vi "Node v1.vi"() -> ()   [LabVIEW 2016]
uses:
  PXImc Router/Controls/Node Data.ctl
  <vilib>/NI Veristand/VeriStand Data/Byte Buffer/Byte Buffer.lvclass
  PXImc Router/Controls/Node/Node - PXImc Parameters.ctl
  PXImc Router/Controls/Node/Node - Writer Data.ctl
  PXImc Router/Controls/Node/Node Ch Properties.ctl
  PXImc Router/Controls/Data Type.ctl
  PXImc Router/Controls/Node/Node - Readers Data.ctl
  PXImc Router/Controls/Node/Node - Reader Data.ctl
  <vilib>/Utility/error.llb/DialogType.ctl
  PXImc Router/VIs/Node/Node - Globals.vi
  PXImc Router/PXImc Router.lvlib
panel:
  in  "Node 2 Data In":T1
  out "Reader Node 2":T8(graph)
  out "Node 2 - Reader Ch":dbl[](array[numeric])
  in  "index 2":i32
  in  "length 2":i32
  out "Writer Node 2":T8(graph)={"[0]"=1.0, "[1]"=2.0, "[2]"=3.0, "[3]"=4.0, "[4]"=5.0, "[5]"=0.0, "[6]"=0.0, "[7]"=0.0, "[8]"=0.0}
  in  "Node 2 - Writer Ch":dbl[](array[numeric])
  in  "length":i32
  in  "index":i32
  out "Node 1 - Reader Ch":dbl[](array[numeric])
  in  "Node 1 Data In":T1
  in  "Node 1 - Writer Ch":dbl[](array[numeric])
  in  "stop":bool
  out "Writer Node 1":T8(graph)={"[0]"=1.0, "[1]"=2.0, "[2]"=3.0, "[3]"=4.0, "[4]"=5.0, "[5]"=0.0, "[6]"=0.0, "[7]"=0.0, "[8]"=0.0}
  out "Reader Node 1":T8(graph)
  # "Node 1"
  # "Node 2"
  # "Node 2 => Node 1"
  # "Node 1 => Node 2"
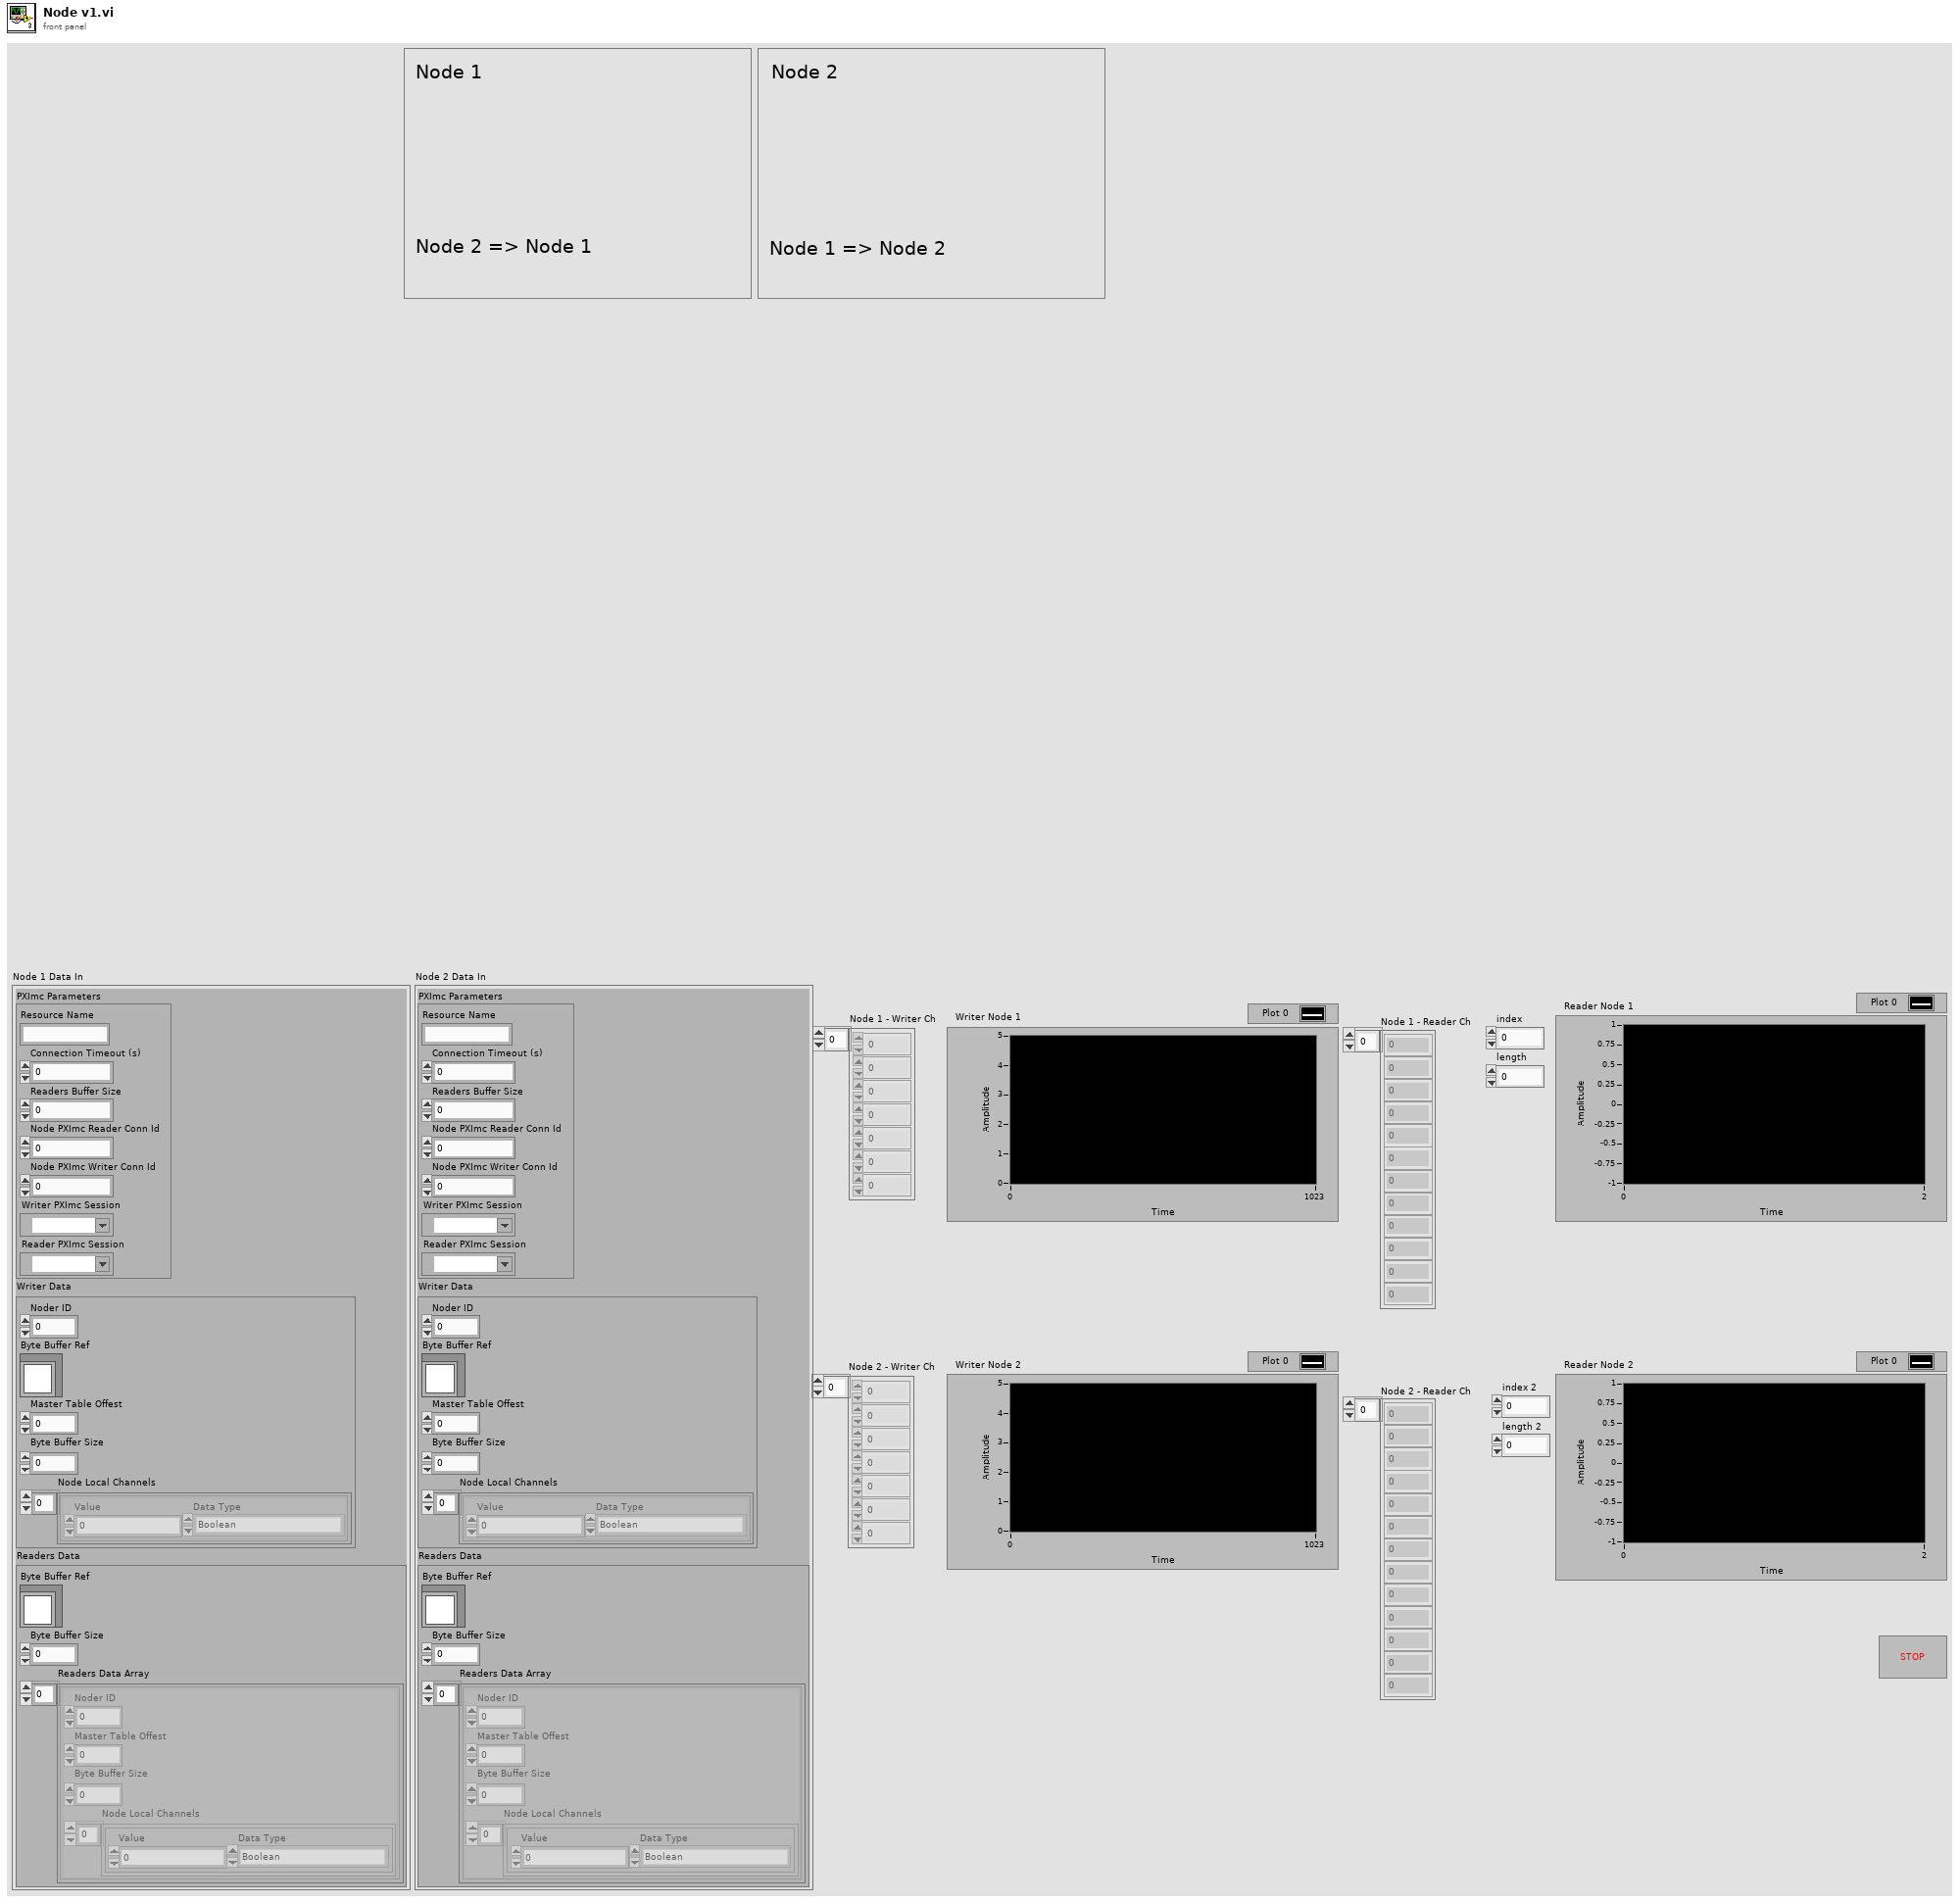
[diagram p1: front panel]
types:
  T1 = typedef "PXImc Router.lvlib/Node Data.ctl" = cluster{"PXImc Parameters":T2, "Writer Data":T3, "Readers Data":T6}
  T2 = typedef "PXImc Router.lvlib/Node - PXImc Parameters.ctl" = cluster{"Resource Name":string, "Connection Timeout (s)":dbl, "Readers Buffer Size":u64, "Node PXImc Reader Conn Id":u16, "Node PXImc Writer Conn Id":u16, "Writer PXImc Session":refnum<k21>, "Reader PXImc Session":refnum<k21>}
  T3 = typedef "PXImc Router.lvlib/Node - Writer Data.ctl" = cluster{"Noder ID":u32, "Byte Buffer Ref":refnum<class "Byte Buffer.lvclass">, "Master Table Offest":u32, "Byte Buffer Size":u32, "Node Local Channels":T4[]}
  T4 = typedef "PXImc Router.lvlib/Node Ch Properties.ctl" = cluster{"Value":dbl, "Data Type":T5}
  T5 = typedef "PXImc Router.lvlib/Data Type.ctl" = enum16{"Boolean", "SGL", "DBL", "I8", "I16", "I32", "I64", "U8", "U16", "U32", "U64"}
  T6 = typedef "PXImc Router.lvlib/Node - Readers Data.ctl" = cluster{"Byte Buffer Ref":refnum<class "Byte Buffer.lvclass">, "Byte Buffer Size":u64, "Readers Data Array":T7[]}
  T7 = typedef "PXImc Router.lvlib/Node - Reader Data.ctl" = cluster{"Noder ID":u32, "Master Table Offest":u32, "Byte Buffer Size":u64, "Node Local Channels":T4[]}
  T8 = cluster{"[0]":dbl, "[1]":dbl, "[2]":dbl, "[3]":dbl, "[4]":dbl, "[5]":dbl, "[6]":dbl, "[7]":dbl, "[8]":dbl}
  T9 = typedef "DialogType.ctl" = u16
  T10 = cluster{"Node 1 - Writer Ch[0]":dbl, "Node 1 - Writer Ch[1]":dbl, "Node 1 - Writer Ch[2]":dbl, "Node 1 - Writer Ch[3]":dbl, "Node 1 - Writer Ch[4]":dbl, "Node 1 - Writer Ch[5]":dbl, "Node 1 - Writer Ch[6]":dbl, "Node 1 - Writer Ch[7]":dbl, "Node 1 - Writer Ch[8]":dbl}
  T11 = cluster{"Node 2 - Writer Ch[0]":dbl, "Node 2 - Writer Ch[1]":dbl, "Node 2 - Writer Ch[2]":dbl, "Node 2 - Writer Ch[3]":dbl, "Node 2 - Writer Ch[4]":dbl, "Node 2 - Writer Ch[5]":dbl, "Node 2 - Writer Ch[6]":dbl, "Node 2 - Writer Ch[7]":dbl, "Node 2 - Writer Ch[8]":dbl}
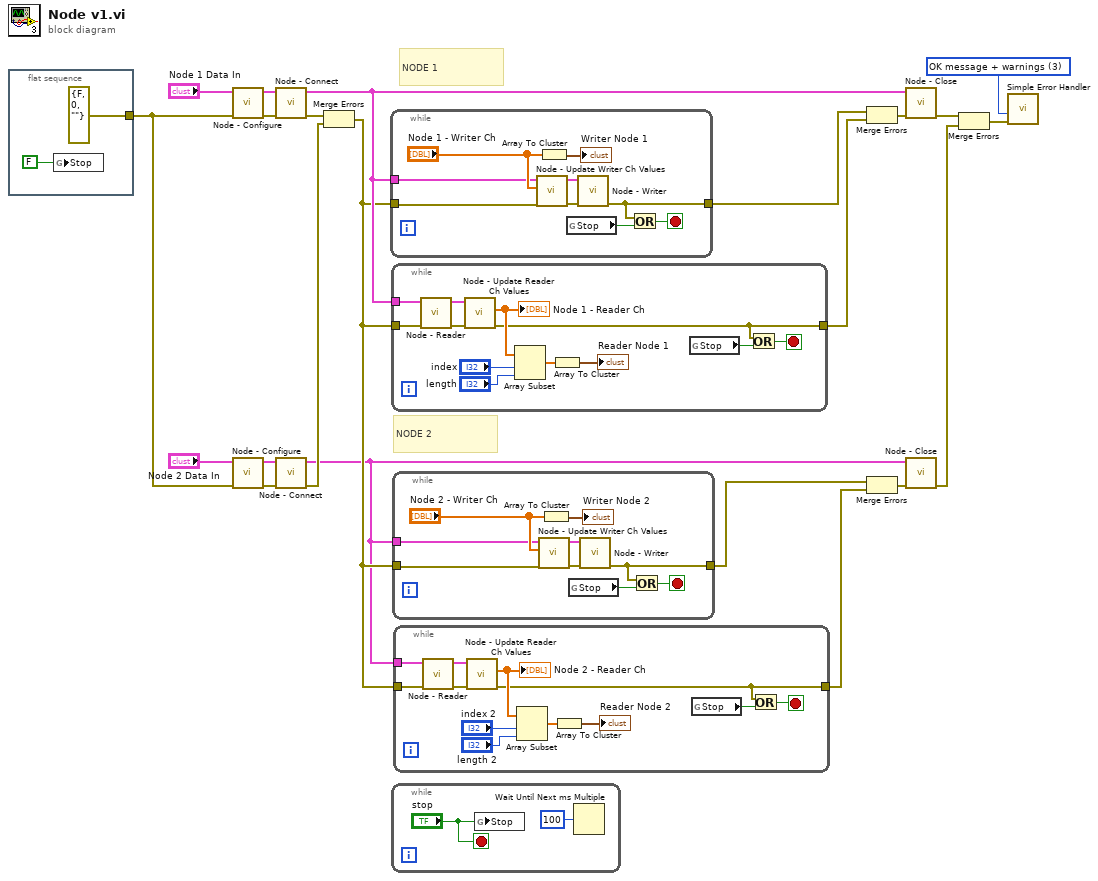
[diagram p0: block diagram]
diagram:
  w22 = T9 3 items=["no dialog", "OK message", "continue or stop message", "OK message + warnings", "continue/stop + warnings"] ("type of dialog (OK msg:1)")
  # "NODE 2"
  # "NODE 1"
  n1 = flat-sequence {
    tunnel: [errorcluster {"status"=FALSE, "code"=0, "source"=""} ("error constant")] -> w6
    frame #0 {
      n2 = global write "Node - Globals.vi" "Stop"(FALSE ("Stopped")) -> ()
    }
  }
  n3 = call "Node - Configure.vi"("error in (no error)"=w6, "Node Data In"="Node 1 Data In") -> ("error out"=w18:errorcluster, "Node Data Out"=w19:T1)  [unwired: 8 in]
  n4 = call "Node - Configure.vi"("error in (no error)"=w6, "Node Data In"="Node 2 Data In") -> ("error out"=w10:errorcluster, "Node Data Out"=w9:T1)  [unwired: 8 in]
  n5 = call "Node - Connect.vi"("error in (no error)"=w18, "Node Data In"=w19) -> ("error out"=w17:errorcluster, "Node Data Out"=w14:T1)  [unwired: 8 in]
  n6 = call "Node - Connect.vi"("error in (no error)"=w10, "Node Data In"=w9) -> ("error out"=w7:errorcluster, "Node Data Out"=w4:T1)  [unwired: 8 in]
  n7 = Merge Errors(w17, w7) -> (w8:errorcluster)
  n8 = while {
    tunnel: w14 -> [w28]
    tunnel: w8 -> [w27]
    tunnel: [w31] -> w21
    stop <- w32 stop-if-true
    n9 = call "Node - Update Writer Ch Values.vi"("error in (no error)"=w27, "Writer Channels In"="Node 1 - Writer Ch", "Node Data In"=w28) -> ("error out"=w25:errorcluster, "Node Data Out"=w26:T1)  [unwired: 7 in]
    n10 = Array To Cluster(array="Node 1 - Writer Ch") -> (cluster=→"Writer Node 1":T10)
    n11 = global read "Node - Globals.vi" "Stop"() -> (w33:bool)
    n12 = call "Node - Writer.vi"("error in (no error)"=w25, "Node Data In"=w26) -> ("error out"=w31:errorcluster)  [unwired: 8 in, 1 out]
    n13 = Or(x=w31, y=w33) -> (x .or. y?=w32:bool)
  }
  n14 = while {
    tunnel: w14 -> [w41]
    tunnel: w8 -> [w45]
    tunnel: [w34] -> w20
    stop <- w43 stop-if-true
    n15 = call "Node - Reader.vi"("error in (no error)"=w45, "Node Data In"=w41) -> ("error out"=w39:errorcluster, "Node Data Out"=w40:T1)  [unwired: 8 in]
    n16 = call "Node - Update Reader Ch Values.vi"("error in (no error)"=w39, "Node Data In"=w40) -> ("error out"=w34:errorcluster, "Reader Ch Out"=w37:dbl[])  [unwired: 7 in, 1 out]
    "Node 1 - Reader Ch" <- w37
    n17 = Array Subset(array=w37, index="index", length="length") -> (w38:dbl[])
    n18 = Array To Cluster(array=w38) -> (cluster=→"Reader Node 1":T8)
    n19 = global read "Node - Globals.vi" "Stop"() -> (w44:bool)
    n20 = Or(x=w34, y=w44) -> (x .or. y?=w43:bool)
  }
  n21 = while {
    stop <- "stop" stop-if-true
    n22 = global write "Node - Globals.vi" "Stop"("stop") -> ()
    n23 = Wait Until Next ms Multiple(millisecond multiple=u32 100) -> ()  [unwired: 1 out]
  }
  n24 = while {
    tunnel: w4 -> [w51]
    tunnel: w8 -> [w50]
    tunnel: [w54] -> w3
    stop <- w55 stop-if-true
    n25 = call "Node - Update Writer Ch Values.vi"("error in (no error)"=w50, "Writer Channels In"="Node 2 - Writer Ch", "Node Data In"=w51) -> ("error out"=w48:errorcluster, "Node Data Out"=w49:T1)  [unwired: 7 in]
    n26 = Array To Cluster(array="Node 2 - Writer Ch") -> (cluster=→"Writer Node 2":T11)
    n27 = global read "Node - Globals.vi" "Stop"() -> (w56:bool)
    n28 = call "Node - Writer.vi"("error in (no error)"=w48, "Node Data In"=w49) -> ("error out"=w54:errorcluster)  [unwired: 8 in, 1 out]
    n29 = Or(x=w54, y=w56) -> (x .or. y?=w55:bool)
  }
  n30 = while {
    tunnel: w4 -> [w64]
    tunnel: w8 -> [w68]
    tunnel: [w57] -> w2
    stop <- w66 stop-if-true
    n31 = call "Node - Reader.vi"("error in (no error)"=w68, "Node Data In"=w64) -> ("error out"=w62:errorcluster, "Node Data Out"=w63:T1)  [unwired: 8 in]
    n32 = call "Node - Update Reader Ch Values.vi"("error in (no error)"=w62, "Node Data In"=w63) -> ("error out"=w57:errorcluster, "Reader Ch Out"=w60:dbl[])  [unwired: 7 in, 1 out]
    "Node 2 - Reader Ch" <- w60
    n33 = Array Subset(array=w60, index="index 2", length="length 2") -> (w61:dbl[])
    n34 = Array To Cluster(array=w61) -> (cluster=→"Reader Node 2":T8)
    n35 = global read "Node - Globals.vi" "Stop"() -> (w67:bool)
    n36 = Or(x=w57, y=w67) -> (x .or. y?=w66:bool)
  }
  n37 = Merge Errors(w21, w20) -> (w16:errorcluster)
  n38 = Merge Errors(w3, w2) -> (w5:errorcluster)
  n39 = call "Node - Close.vi"("error in (no error)"=w16, "Node Data In"=w14) -> ("error out"=w15:errorcluster)  [unwired: 9 in]
  n40 = call "Node - Close.vi"("error in (no error)"=w5, "Node Data In"=w4) -> ("error out"=w1:errorcluster)  [unwired: 9 in]
  n41 = Merge Errors(w15, w1) -> (w13:errorcluster)
  n42 = call <vilib>:"Simple Error Handler.vi"("type of dialog (OK msg:1)"=w22, "error in (no error)"=w13) -> ()  [unwired: 3 in, 5 out]
